vi "getMode.vi"(8 "error in (no error)":errorcluster, 11 "DmmKeysight in":refnum<class "DmmKeysight.lvclass">) -> (0 "error out":errorcluster, 2 "mode":T1, 3 "DmmKeysight out":refnum<class "DmmKeysight.lvclass">)   [LabVIEW 2023, in "DmmKeysight.lvclass"]
doc: "<b>Author:</b> Wolfgang\n<b>Description:</b>Query Dmm for measurement mode: Voltage, Current, Resistance"
uses:
  DmmKeysight.lvclass
  Data/DmmModes.ctl
  DmmKeysight.lvclass/DmmKeysight.ctl
  sweDmm.lvlib
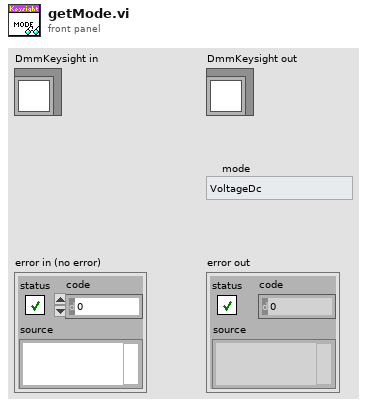
[diagram p1: front panel]
types:
  T1 = typedef "sweDmm.lvlib/DmmModes.ctl" = enum16{"VoltageDc", "VoltageAc", "CurrentDc", "CurrentAc", "Resistance2W"}
  T2 = typedef "Keysight-34450A.lvlib/mode.ctl" = enum16{"DC_Voltage", "AC_Voltage", "DC_Current", "AC_Current", "Resistance"}
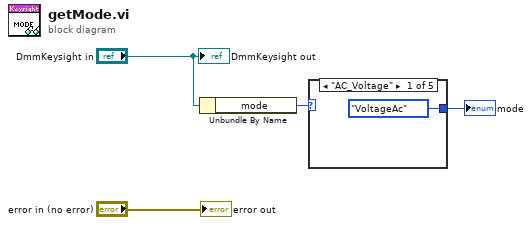
[diagram p0: block diagram]
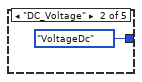
[diagram p2: hidden frame]
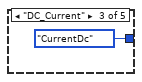
[diagram p3: hidden frame]
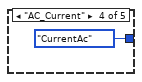
[diagram p4: hidden frame]
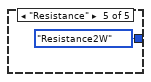
[diagram p5: hidden frame]
diagram:
  n1 = Unbundle By Name("DmmKeysight in") -> ("mode"=w2:T2)
  n2 = case shown="\"AC_Voltage\"" w2 {
    tunnel: [DmmModes."VoltageAc" ("mode") DmmModes."VoltageDc" ("mode") DmmModes."CurrentDc" ("mode") DmmModes."CurrentAc" ("mode") DmmModes."Resistance2W" ("mode")] -> w1
    frame "AC_Voltage" {
    }
    frame "DC_Voltage" {
    }
    frame "DC_Current" {
    }
    frame "AC_Current" {
    }
    frame "Resistance" {
    }
  }
  "mode" <- w1
  "error out" <- "error in (no error)"
  "DmmKeysight out" <- "DmmKeysight in"
